vi "clLabview_LVSR.vi"(0 "vi_lib.lvlib:clLabview.lvclass":refnum<class "clLabview.lvclass">) -> (6 "major":u8=3 min=1 max=99 step=1, 7 "(unknown) INT1":i32 step=1, 8 "minor":u8 max=99 step=1, 9 "File Flags":i32 step=1, 10 "bugfix":u8 step=1, 12 "build":u8 step=1, 14 "stage":u8(ring) items=["development", "alpha", "beta", "release"], 17 "File is protected?":bool=TRUE, 18 "MD5 lib Password":string, 19 "MD5 lib Password (Hex)":string)   [LabVIEW 2021, in "vi_lib.lvlib" / "clLabview.lvclass"]
uses:
  clLabview.lvclass
  clFileReader/clFileReader.lvclass
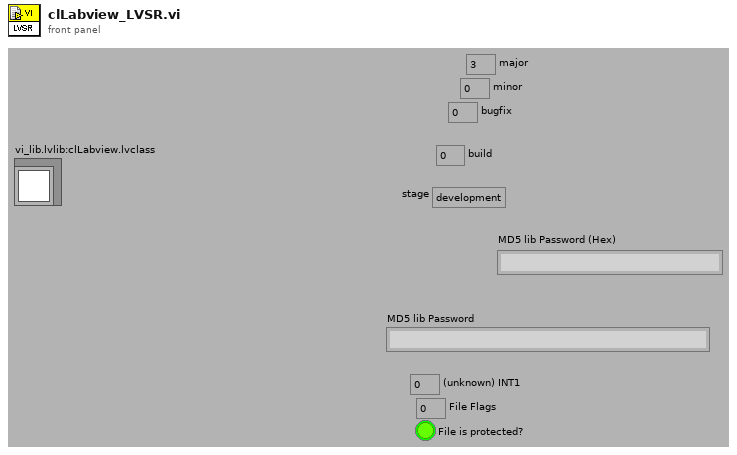
[diagram p1: front panel]
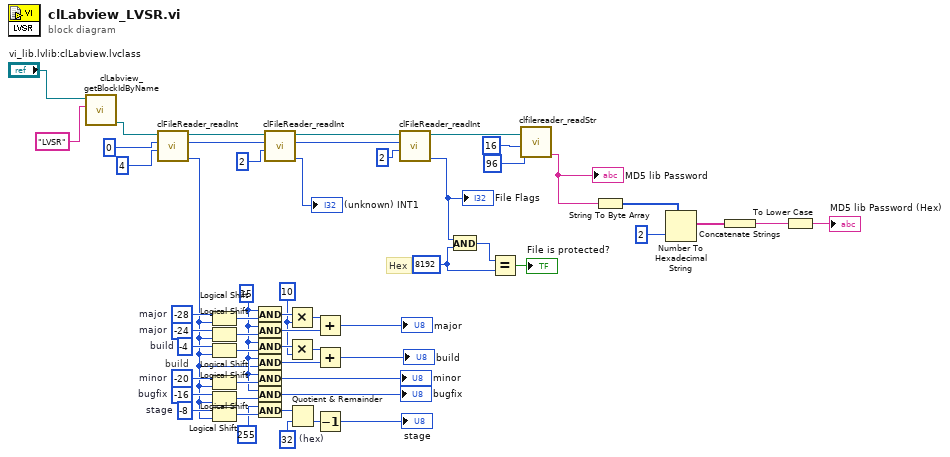
[diagram p0: block diagram]
diagram:
  w8 = u32 8192
  w33 = 32  # (hex)
  w43 = 15
  w44 = i8 -4  # build
  w45 = i8 -8  # stage
  w46 = i8 -16  # bugfix
  w47 = i8 -20  # minor
  w48 = i8 -24  # major
  w49 = i8 -28  # major
  w34 = 10
  # "Hex"
  # "build"
  n1 = call "clLabview_getBlockIdByName.vi"("Block Name"="LVSR", "vi_lib.lvlib:clLabview.lvclass"="vi_lib.lvlib:clLabview.lvclass") -> ("Block Content"=w24:refnum<class "clFileReader.lvclass">)  [unwired: 2 in, 6 out]
  n2 = call "clFileReader_readInt.vi"("size"=u32 4, "offset"=u32 0, "clFileReader.lvclass IN"=w24) -> ("OUT Value"=w21:u32, "new offset"=w20:u32, "clFileReader.lvclass OUT"=w17:refnum<class "clFileReader.lvclass">)  [unwired: 6 out]
  n3 = Logical Shift(y=w49, x=w21) -> (x << y=w55:u32)
  n4 = Logical Shift(y=w48, x=w21) -> (x << y=w54:u32)
  n5 = Logical Shift(y=w44, x=w21) -> (x << y=w50:u32)
  n6 = Logical Shift(y=w47, x=w21) -> (x << y=w53:u32)
  n7 = Logical Shift(y=w46, x=w21) -> (x << y=w52:u32)
  n8 = Logical Shift(y=w45, x=w21) -> (x << y=w51:u32)
  n9 = And(x=w43, y=w55) -> (x .and. y?=w37:u32)
  n10 = And(x=w43, y=w54) -> (x .and. y?=w40:u32)
  n11 = And(x=w43, y=w50) -> (x .and. y?=w36:u32)
  n12 = And(x=w43, y=w21) -> (x .and. y?=w38:u32)
  n13 = And(x=w43, y=w53) -> (x .and. y?=→"minor":u32)
  n14 = And(x=w43, y=w52) -> (x .and. y?=→"bugfix":u32)
  n15 = And(x=255, y=w51) -> (x .and. y?=w35:u32)
  n16 = call "clFileReader_readInt.vi"("size"=u32 2, "offset"=w20, "clFileReader.lvclass IN"=w17) -> ("OUT Value"=→"(unknown) INT1":u32, "new offset"=w15:u32, "clFileReader.lvclass OUT"=w16:refnum<class "clFileReader.lvclass">)  [unwired: 6 out]
  n17 = Multiply(x=w37, y=w34) -> (x*y=w41:u32)
  n18 = Multiply(x=w36, y=w34) -> (x*y=w39:u32)
  n19 = Quotient & Remainder(x=w35, y=w33) -> (floor(x/y)=w32:u32)  [unwired: 1 out]
  n20 = Add(x=w41, y=w40) -> (x+y=→"major":u32)
  n21 = Add(x=w39, y=w38) -> (x+y=→"build":u32)
  n22 = Decrement(x=w32) -> (x-1=→"stage":u32)
  n23 = call "clFileReader_readInt.vi"("size"=u32 2, "offset"=w15, "clFileReader.lvclass IN"=w16) -> ("OUT Value"=w10:u32, "clFileReader.lvclass OUT"=w13:refnum<class "clFileReader.lvclass">)  [unwired: 7 out]
  "File Flags" <- w10
  n24 = And(x=w10, y=w8) -> (x .and. y?=w9:u32)
  n25 = Equal?(x=w9, y=w8) -> (x = y?=→"File is protected?":bool)
  n26 = call "clfilereader_readStr.vi"("size"=u32 16, "offset"=u32 96, "clFileReader.lvclass IN"=w13) -> ("ReadStr - OUT Value"=w1:string)  [unwired: 8 out]
  "MD5 lib Password" <- w1
  n27 = String To Byte Array(string=w1) -> (unsigned byte array=w6:u8[])
  n28 = Number To Hexadecimal String(1:i16 2 ("width (-)"), 2:w6) -> (0:w4:string[])
  n29 = Concatenate Strings(w4) -> (w3:string)
  n30 = To Lower Case(string=w3) -> (all lower case string=→"MD5 lib Password (Hex)":string)
